vi "PH_ImageOperator.PC set Trace Analysis.vi"(0 "i ref in":refnum<vi>, 2 "Trace Analysis on":bool, 5 "error in (no error)":errorcluster) -> (14 "i ref out":refnum<vi>, 19 "error out":errorcluster)   [LabVIEW 2014, in "PH_ImageOperator.lvlib"]
doc: "This is the action of the \"SetTraceAnalOn\"."
uses:
  PH_ImageOperator.lvlib
  CSCore/CSSystem/CSSystemLib/CSSystemLib.lvlib
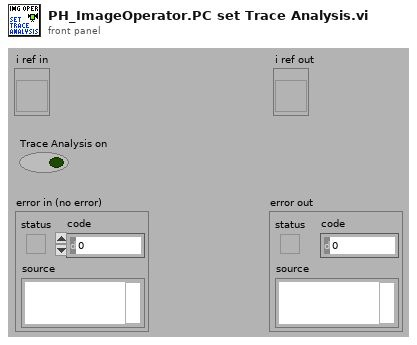
[diagram p1: front panel]
types:
  T1 = typedef "PH_ImageOperator.lvlib/PH_ImageOperator.i attribute.ctl" = cluster{"GUI Refs":cluster{"Delete":refnum<vi>, "Calibration status":refnum<vi>, "BI subtracted":refnum<vi>, "calc Energy":refnum<vi>, "Energy: expected value":refnum<vi>, "Energy: Tolerance":refnum<vi>, "Energy calculated":refnum<vi>, "Energy":refnum<vi>, "calc Beam Anal":refnum<vi>, "Maj Diam 1/esquare":refnum<vi>, "Min Diam 1/esquare":refnum<vi>, "Azi Angle":refnum<vi>, "Min/Maj Diam esquare":refnum<vi>, "Beam analysed":refnum<vi>, "CoG - x":refnum<vi>, "CoG - y":refnum<vi>, "BA: Method":refnum<vi>, "BA: Steps":refnum<vi>, "BA: Factor":refnum<vi>, "calc Traces":refnum<vi>, "Traces: Fit Gauss":refnum<vi>, "Traces calculated":refnum<vi>, "Maj FWHM":refnum<vi>, "Min FWHM":refnum<vi>, "Major Trace":refnum<vi>, "Minor Trace":refnum<vi>, "Maj Fit Order":refnum<vi>, "Min Fit Order":refnum<vi>, "Position calculated":refnum<vi>, "Position":refnum<vi>, "Type":refnum<vi>, "Center":refnum<vi>, "exp - X":refnum<vi>, "exp - Y":refnum<vi>, "Tolerance":refnum<vi>, "f":refnum<vi>, "M":refnum<vi>, "D":refnum<vi>, "q":refnum<vi>, "Dummy Method":refnum<vi>, "Dummy Type":refnum<vi>, "Global On":refnum<vi>, "Traces: No offset":refnum<vi>, "Maj 99%":refnum<vi>, "Min 99%":refnum<vi>, "GUI FF Image":refnum<vi>, "calc Fill Factor":refnum<vi>, "FF calculated":refnum<vi>, "Fill Factor: Filter?":refnum<vi>, "FF: Damage Threshold":refnum<vi>, "FF: Threshold":refnum<vi>, "FF: max allow. Energy":refnum<vi>, "FF: Fillfactor":refnum<vi>, "Calibration data":refnum<vi>}, "List of GUIs":string[], "Calibration":cluster{"Status":T2, "Calibration data":T3, "Calibration Data File":path}, "Final Image":cluster{"BI Subtraction Failure":bool}, "Energy":cluster{"on":bool, "expected value [mJ]":dbl, "Tolerance [%]":dbl, "State":T2, "Energy [mJ]":dbl, "Unit":string, "calculated @":timestamp}, "Beam Analysis":cluster{"on":bool, "Data":T4, "Method":bool, "Steps":i32, "Factor":i32, "ROI":cluster{"Left":i32, "Top":i32, "Right":i32, "Bottom":i32}, "analysed @":timestamp}, "Trace Analysis":cluster{"on":bool, "Fit on":bool, "Maj FWHM":dbl, "Min FWHM":dbl, "Maj Fit Order":i32, "Min Fit Order":i32, "No Offset":bool, "Maj 99%":dbl, "Min 99%":dbl, "Traces":cluster{"XScaleName":string, "Y Scale Minimum":sgl, "Y Scale Maximum":sgl, "X Scale Minimum":sgl, "X Scale Maximum":sgl, "Traces":cluster{"Index":sgl[], "Trace":dbl[]}[]}[], "analysed @":timestamp}, "Position Analysis":cluster{"on":bool, "exp - X":i32, "exp - Y":i32, "focal length [mm]":dbl, "Magnification":dbl, "Delta":dbl, "Theta":dbl, "Tolerance":dbl, "Type":bool, "analysed @":timestamp}, "Fill Factor":cluster{"on":bool, "Filter on?":bool, "Threshold":dbl, "Damage Threshold [J/cm²]":dbl, "Fillfactor":dbl, "Max. allowed Energy [J]":dbl, "calculated @":timestamp}, "Statistician Service ID":i32, "Images":cluster{"Background":T5, "OP":T5, "GUI":T5, "BA: ROI":T5, "Trace: Turn":T5, "FF: Main":T5, "FF: Help":T5, "PSDB: BG":T5, "PSDB: OP":T5, "PSDB: FF":T5}}
  T2 = typedef "PH_StatusHandler.lvlib/PH_StatusHandler.Status.ctl" = i16
  T3 = typedef "PH_ImageCalibrator.lvlib/PH_ImageCalibrator.Calibration Data.ctl" = cluster{"Date":string, "Time":string, "Cam Settings":cluster{"Cam ID":string, "Gain":dbl, "Brightness":dbl, "Shutter":dbl, "Cam Error":bool, "Mode":i32}, "Background Image":cluster{"Image":dbl[][], "Image Error":bool}, "Linear Calibration":cluster{"Calibration Factor":dbl, "not mm or mrad":bool}, "Energy Calibration":cluster{"Calibration Factor":dbl, "no mJ":bool}}
  T4 = typedef "PH_ImageOperator.lvlib/PH_ImageOperator.Beam Analysis Data.ctl" = cluster{"CoG-x":sgl, "CoG-y":sgl, "Maj Dim":dbl, "Min Dim":dbl, "Ellipticity":dbl, "Azimuth Angle [rad]":dbl, "Azi Angle rel to Maj?":bool}
  T5 = typedef "IMAQ Image.ctl" = refnum<image>
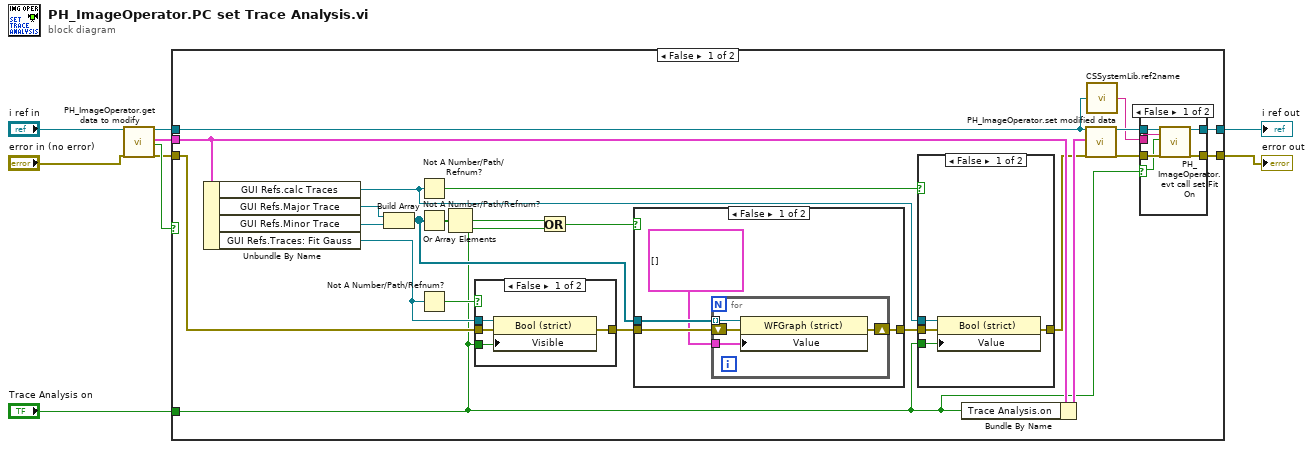
[diagram p0: block diagram]
diagram:
  n1 = call "PH_ImageOperator.get data to modify.vi"("i ref in"="i ref in", "error in (no error)"="error in (no error)") -> ("i ref out"=w4:refnum<vi>, "i attribute"=w8:T1, "timed out"=w7:bool, "error out"=w1:errorcluster)  [unwired: 14 in]
  n2 = case shown="False" w7 {
    tunnel: w1 -> [w28 w60]
    tunnel: [w15 w60] -> w3
    tunnel: w4 -> [w13 w61]
    tunnel: [w14 w61] -> w6
    tunnel: w8 -> [w31 _]
    tunnel: "Trace Analysis on" -> [w10 _]
    frame False {
      n3 = Unbundle By Name(w31) -> ("GUI Refs.calc Traces"=w21:refnum<vi>, "GUI Refs.Major Trace"=w24:refnum<vi>, "GUI Refs.Minor Trace"=w25:refnum<vi>, "GUI Refs.Traces: Fit Gauss"=w18:refnum<vi>)
      n4 = Build Array(w24, w25) -> (w22:refnum<vi>[])
      n5 = Not A Number/Path/Refnum?(number/path/refnum=w21) -> (NaN/Path/Refnum?=w29:bool)
      n6 = Not A Number/Path/Refnum?(number/path/refnum=w22) -> (NaN/Path/Refnum?=w23:bool[])
      n7 = Not A Number/Path/Refnum?(number/path/refnum=w18) -> (NaN/Path/Refnum?=w17:bool)
      n8 = Or Array Elements(Boolean array=w23) -> (logical OR=w20:bool)
      n9 = case shown="False" w17 {
        tunnel: w10 -> [w53 _]
        tunnel: w28 -> [w52 w54]
        tunnel: [w51 w54] -> w27
        tunnel: w18 -> [w50 _]
        frame False {
          n10 = property class="Bool (strict)"(reference=w50, error in=w52, "Visible"=w53) -> (error out=w51:errorcluster)  [unwired: 1 out]
        }
        frame True {
        }
      }
      n11 = Or(x=w20, y=w10) -> (x .or. y?=w19:bool)
      n12 = case shown="False" w19 {
        tunnel: w27 -> [w44 w49]
        tunnel: [w43 w49] -> w26
        tunnel: w22 -> [w42 _]
        frame False {
          n13 = for {
            tunnel: w42 -> [w46] mode=indexing
            shift-right: [w47] -> w43
            shift-left: w44 -> [w48]
            tunnel: cluster{"Index":sgl[], dbl[]}[] [] ("Value") -> [w45]
            n14 = property class="WFGraph (strict)"(reference=w46, error in=w48, "Value"=w45) -> (error out=w47:errorcluster)  [unwired: 1 out]
          }
        }
        frame True {
        }
      }
      n15 = case shown="False" w29 {
        tunnel: w10 -> [w58 _]
        tunnel: w26 -> [w57 w59]
        tunnel: [w56 w59] -> w30
        tunnel: w21 -> [w55 _]
        frame False {
          n16 = property class="Bool (strict)"(reference=w55, error in=w57, "Value"=w58) -> (error out=w56:errorcluster)  [unwired: 1 out]
        }
        frame True {
        }
      }
      n17 = Bundle By Name(cluster=w31, "Trace Analysis.on"=w10) -> (w32:T1)
      n18 = call "PH_ImageOperator.set modified data.vi"("i ref in"=w13, "i attribute"=w32, "error in (no error)"=w30) -> ("i ref out"=w12:refnum<vi>, "error out"=w16:errorcluster)  [unwired: 15 in]
      n19 = call "CSSystemLib.ref2name.vi"("obj refnum"=w13) -> ("name"=w11:string)
      n20 = case shown="False" w10 {
        selector: w10 -> [w33 _]
        tunnel: w16 -> [w38 w39]
        tunnel: [w37 w39] -> w15
        tunnel: [w36 w40] -> w14
        tunnel: w12 -> [w35 w40]
        tunnel: w11 -> [w34 _]
        frame False {
          n21 = call "PH_ImageOperator.evt call set Fit On.vi"("i ref in"=w35, "Instance"=w34, "Fit on"=w33, "error in (no error)"=w38) -> ("i ref out"=w36:refnum<vi>, "error out"=w37:errorcluster)  [unwired: 14 in]
        }
        frame True {
        }
      }
    }
    frame True {
    }
  }
  "i ref out" <- w6
  "error out" <- w3
